vi "get&set kV&mA.vi"(8 "error in (no error)":errorcluster, 10 "meta info":refnum<k24>, 11 "VGS_MetaInfo in":refnum<class "VGS_MetaInfo.lvclass">) -> (0 "error out":errorcluster, 3 "VGS_MetaInfo out":refnum<class "VGS_MetaInfo.lvclass">)   [LabVIEW 2022 SP3, in "LV_VGS.lvlib" / "VGS_MetaInfo.lvclass"]
uses:
  VGS_MetaInfo.lvclass
  C:/Users/Andrey/Documents/GitHub/LV_VGS/vgs_project.dll
  vgs_project.dll
  VGS_MetaInfo.lvclass/VGS_MetaInfo.ctl
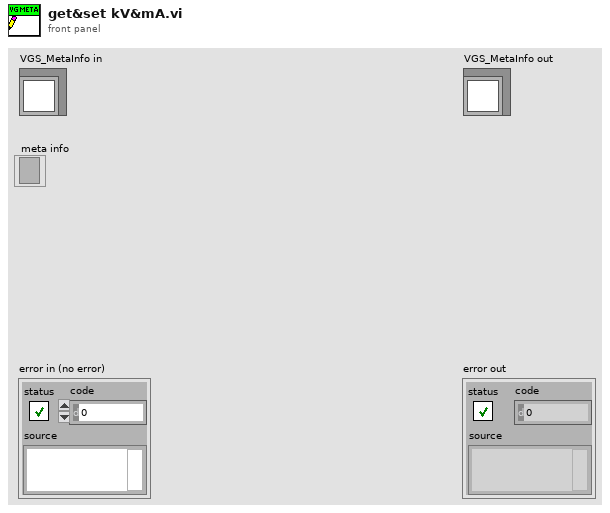
[diagram p1: front panel]
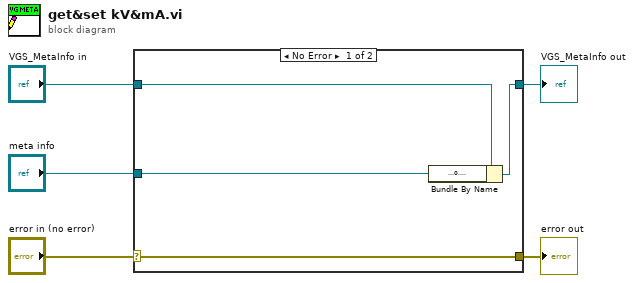
[diagram p0: block diagram]
diagram:
  n1 = case shown="No Error" "error in (no error)" {
    selector: "error in (no error)" -> [w9 w10]
    tunnel: [w9 w10] -> w4
    tunnel: [w7 w11] -> w2
    tunnel: "VGS_MetaInfo in" -> [w8 w11]
    tunnel: "meta info" -> [w6 _]
    frame No Error {
      n2 = Bundle By Name(cluster=w8, "meta info"=w6) -> (w7:refnum<class "VGS_MetaInfo.lvclass">)
    }
    frame Error {
    }
  }
  "error out" <- w4
  "VGS_MetaInfo out" <- w2
